vi "FPGA FIFO Read.vi"(9 "data queue in":refnum<queue>, 11 "FPGA VI Reference In":refnum<k20>) -> ()   [LabVIEW 2018]
uses:
  <vilib>/rvi/interface/nirviMethod/nirviMethod.xnode
  <vilib>/FPGAPlugInAG/Dynamic/niLvFpga_ReadFifo_Dynamic.vi
  <vilib>/rvi/errors/niLvFpgaMergeErrorWithErrorCode.vi
  <vilib>/FPGAPlugInAG/Dynamic/niLvFpga_StartFifo_Dynamic.vi
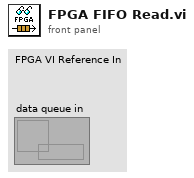
[diagram p1: front panel]
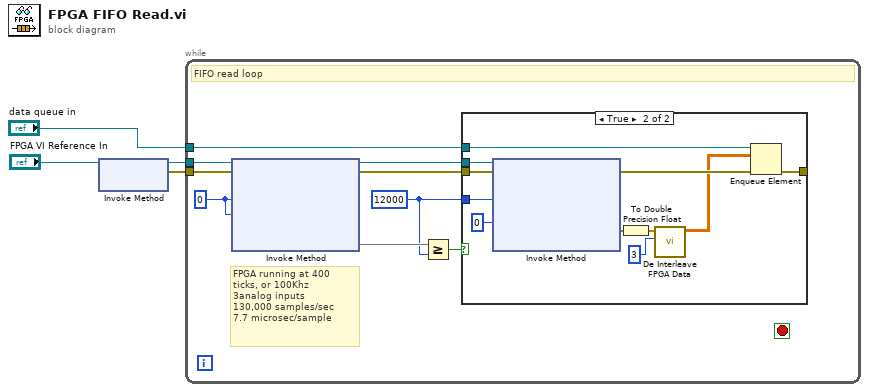
[diagram p0: block diagram]
diagram:
  n1 = xnode "Invoke Method"("FPGA VI Reference In"="FPGA VI Reference In") -> ("FPGA VI Reference Out"=w4:refnum<k20>, "error out"=w3:errorcluster)  [unwired: 1 in]
  n2 = while {
    tunnel: w4 -> [w13]
    tunnel: w3 -> [w7]
    tunnel: "data queue in" -> [w5]
    stop <- _ stop-if-true
    w10 = u32 12000 ("Number of Elements 2")
    w6 = u32 0 ("Number of Elements")
    # "FPGA running at 400 ticks, or 100Khz\n3analog inputs\n130,000 samples/sec\n7.7 microsec/sample"
    # "FIFO read loop"
    n3 = xnode "Invoke Method"("FPGA VI Reference In"=w13, "error in"=w7, "Number of Elements"=w6, "Timeout (ms)"=w6) -> ("FPGA VI Reference Out"=w9:refnum<k20>, "error out"=w8:errorcluster, "Elements Remaining"=w11)  [unwired: 1 out]
    n4 = Greater Or Equal?(x=w11, y=w10) -> (x >= y?=w12:bool)
    n5 = case shown="True" w12 {
      tunnel: w10 -> [_ w25]
      tunnel: w9 -> [_ w22]
      tunnel: w8 -> [w14 w21]
      tunnel: [w14 w19] -> _
      tunnel: w5 -> [_ w15]
      frame False {
      }
      frame True {
        n6 = xnode "Invoke Method"("FPGA VI Reference In"=w22, "error in"=w21, "Number of Elements"=w25, "Timeout (ms)"=0) -> ("error out"=w20:errorcluster, "Data"=w23:void[])  [unwired: 2 out]
        n7 = To Double Precision Float(number=w23) -> (double precision float=w17:dbl[])
        n8 = call "De Interleave FPGA Data.vi"("Number of Interleaved Channels"=u32 3, "Interleaved Data"=w17) -> ("De-Interleaved Channel Data"=w16:dbl[][])  [unwired: 9 in]
        n9 = Enqueue Element(queue=w15, element=w16, error in (no error)=w20) -> (error out=w19:errorcluster)  [unwired: 1 in, 2 out]
      }
    }
  }
